vi "Gyro Signal 3-Axis Display from other MCU.vi"() -> ()   [LabVIEW 2015]
uses:
  <vilib>/Utility/error.llb/DialogType.ctl
  <vilib>/Instr/_visa.llb/VISA Configure Serial Port (Instr).vi
panel:
  out "System Time":dbl
  in  "Stop Button":bool
  out "Z-Array":dbl[](array[numeric])
  out "Y-Array":dbl[](array[numeric])
  out "X-Array":dbl[](array[numeric])
  out "Gyro Reading Z":dbl(knob) scale=-250.0..250.0
  out "Gyro Reading Y":dbl(knob) scale=-250.0..250.0
  out "Data Buffer":u8[](array[numeric])
  in  "parity (0:none)":enum16{"None", "Odd", "Even", "Mark", "Space"}(ring)
  out "Gyro Reading X":dbl(knob) scale=-250.0..250.0
  in  "VISA resource name":refnum<visa-resource-name>="COM5"
  in  "Stop bits (1 bit)":u16(ring)=10 items=["1.0"=10, "1.5"=15, "2.0"=20]
  in  "Baud rate":u32=115200
  # "Setup of Basic Serial Coms"
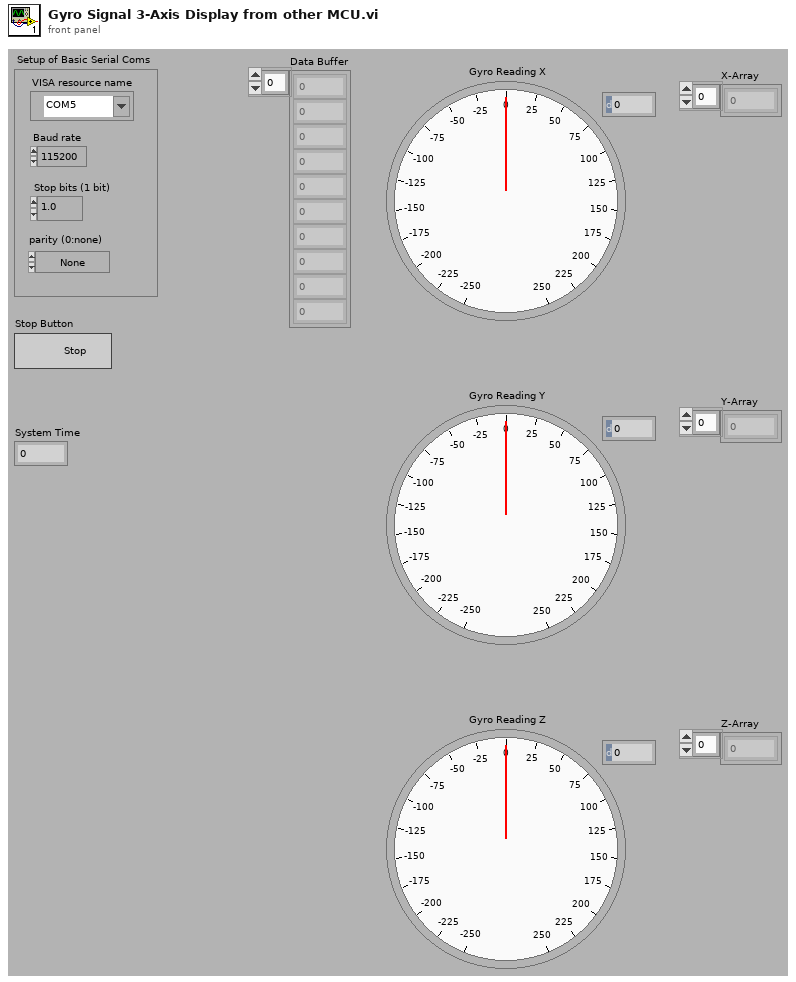
[diagram p1: front panel]
types:
  T1 = typedef "DialogType.ctl" = u16
  T2 = cluster{"Data Buffer[0]":u8, "Data Buffer[1]":u8, "Data Buffer[2]":u8, "Data Buffer[3]":u8, "Data Buffer[4]":u8, "Data Buffer[5]":u8, "Data Buffer[6]":u8, "Data Buffer[7]":u8, "Data Buffer[8]":u8, "Data Buffer[9]":u8}
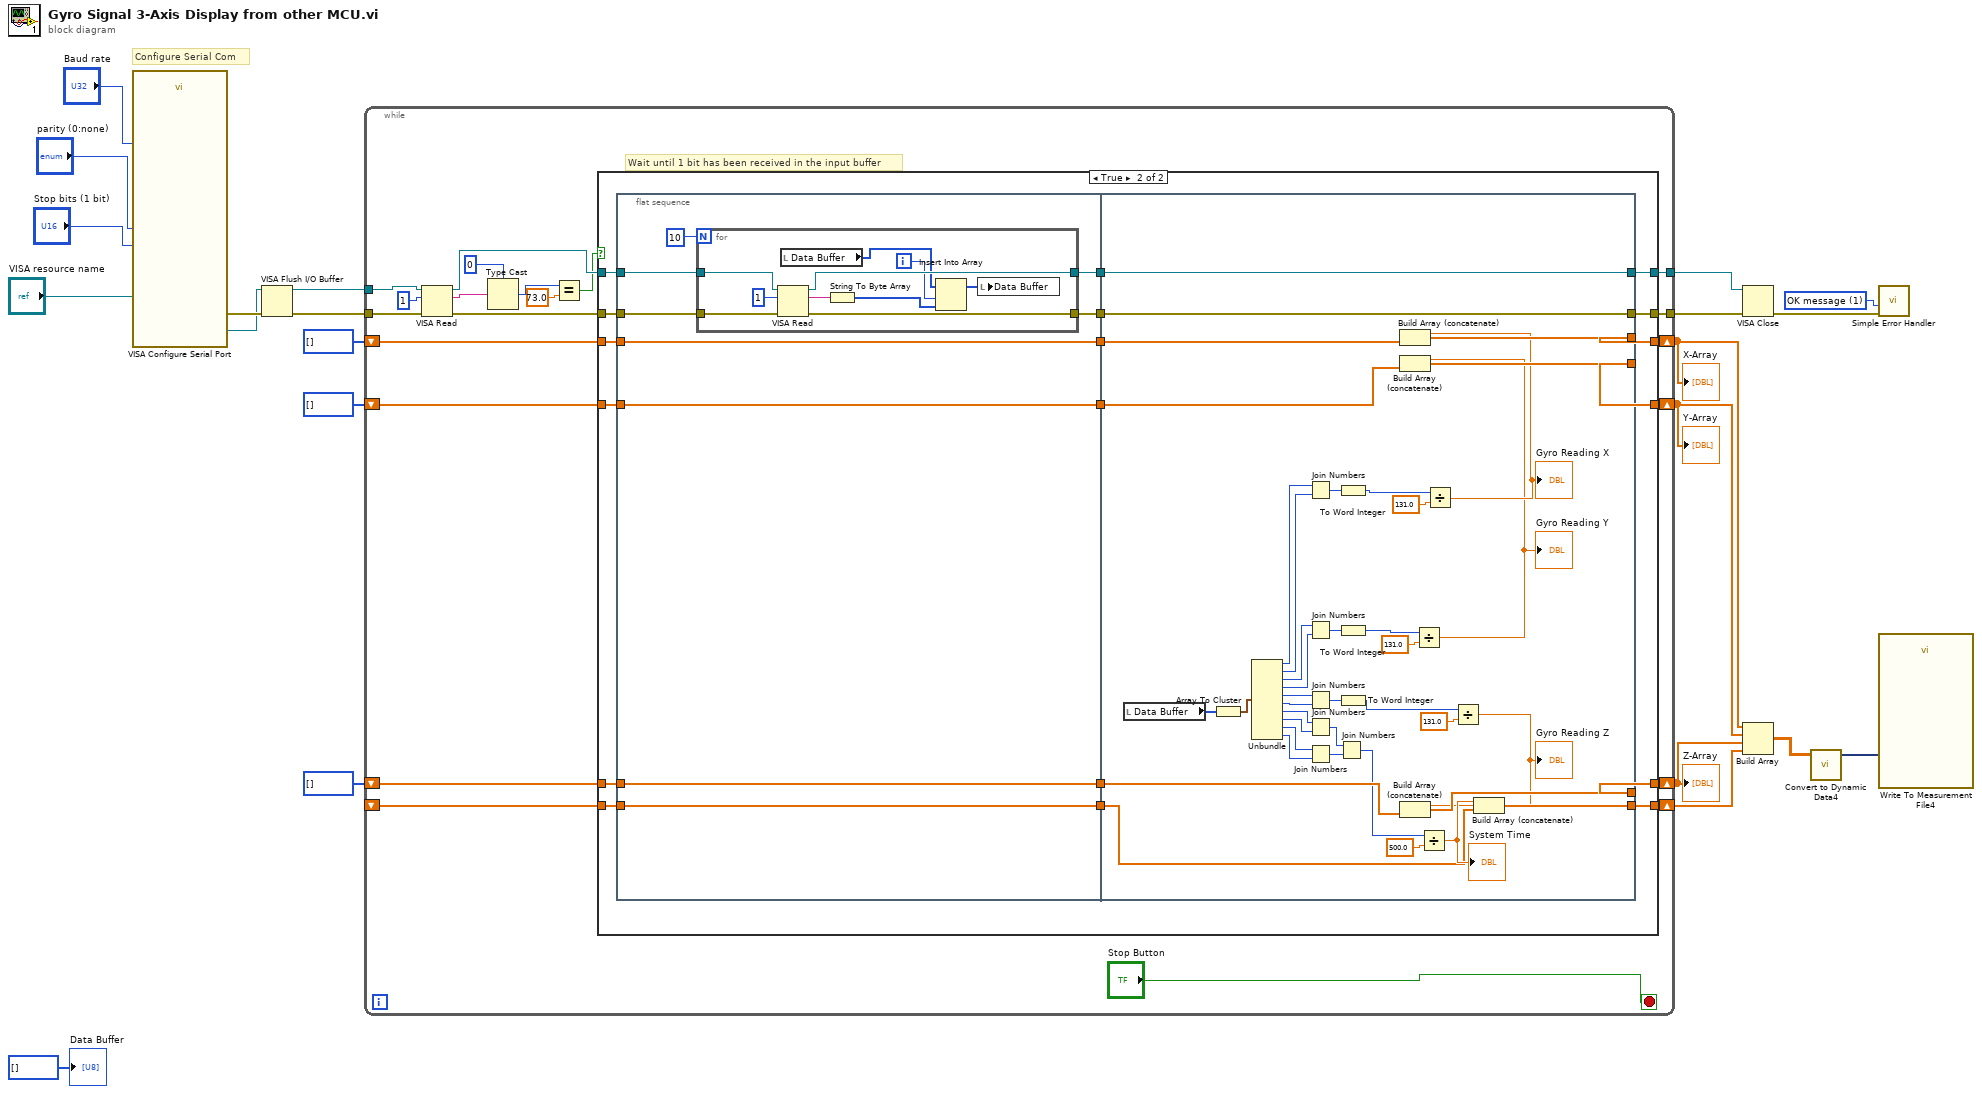
[diagram p0: block diagram]
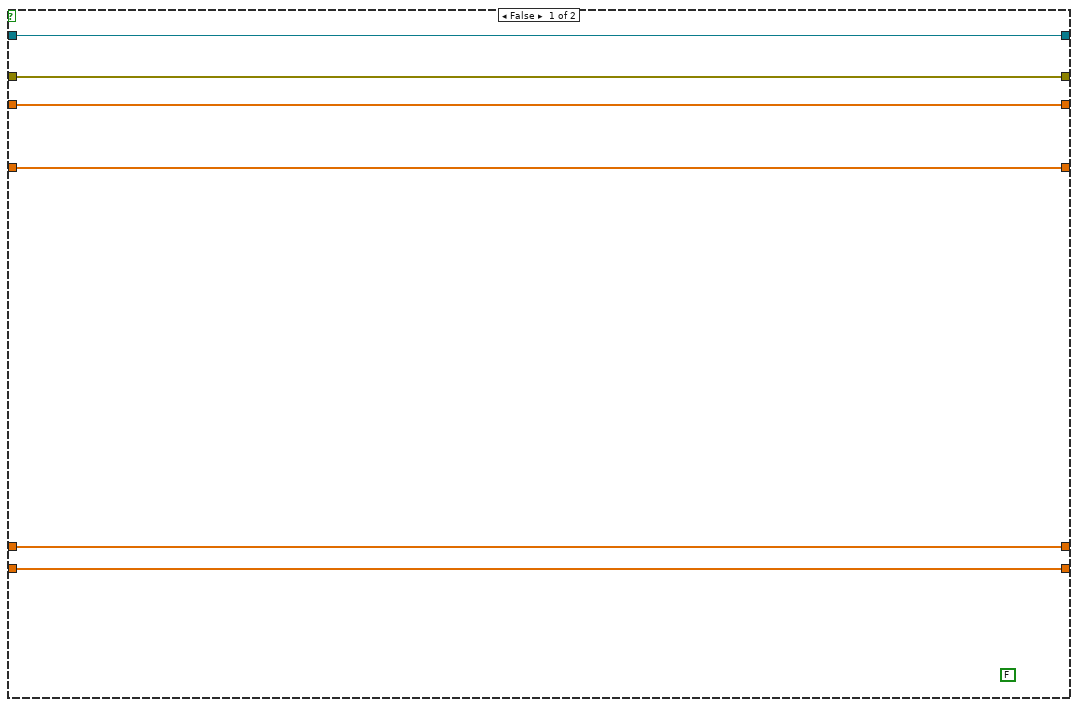
[diagram p2: hidden frame]
diagram:
  w18 = T1 1 items=["no dialog", "OK message", "continue or stop message", "OK message + warnings", "continue/stop + warnings"] ("type of dialog (OK msg:1)")
  # "Configure Serial Com"
  n1 = call-poly "VISA Configure Serial Port"("VISA resource name"="VISA resource name", "baud rate (9600)"="Baud rate", "parity (0:none)"="parity (0:none)", "stop bits (10: 1 bit)"="Stop bits (1 bit)") -> ("VISA resource name out"=w16:refnum<visa-resource-name>, "error out"=w17:errorcluster)  [unwired: 10 in]
  n2 = VISA Flush I/O Buffer(VISA resource name=w16, error in (no error)=w17) -> (VISA resource name out=w15:refnum<visa-resource-name>, error out=w14:errorcluster)  [unwired: 1 in]
  n3 = while {
    tunnel: w15 -> [w35]
    tunnel: w14 -> [w34]
    tunnel: [w43] -> w12
    tunnel: [w42] -> w11
    shift-right: [w41] -> w4
    shift-left: i16[] [] -> [w40]
    shift-right: [w36] -> w3
    shift-left: i16[] [] -> [w37]
    shift-right: [w39] -> w2
    shift-left: i16[] [] -> [w38]
    shift-right: [w25] -> w1
    shift-left: _ -> [w24]
    stop <- "Stop Button" stop-if-true
    # "Wait until 1 bit has been received in the input buffer"
    n4 = VISA Read(VISA resource name=w35, byte count=u32 1, error in (no error)=w34) -> (VISA resource name out=w32:refnum<visa-resource-name>, read buffer=w26:string, error out=w31:errorcluster)  [unwired: 1 out]
    n5 = Type Cast(type=u8 0, x=w26) -> (*(type *) &x=w29:u8)
    n6 = Equal?(x=w29, y=73.0) -> (x = y?=w27:bool)
    n7 = case shown="True" w27 {
      tunnel: [w46 w65] -> w43
      tunnel: [w45 w64] -> w42
      tunnel: [w49 w63] -> w41
      tunnel: w40 -> [w49 w62]
      tunnel: [w48 w60] -> w39
      tunnel: w38 -> [w48 w59]
      tunnel: w37 -> [w47 w57]
      tunnel: [w47 w55] -> w36
      tunnel: w32 -> [w46 w54]
      tunnel: w31 -> [w45 w53]
      tunnel: [w44 w52] -> w25
      tunnel: w24 -> [w44 w51]
      frame False {
        (unwired) FALSE ("LIMIT ERROR")
      }
      frame True {
        n8 = flat-sequence {
          tunnel: [w75] -> w67
          tunnel: [w74] -> w66
          tunnel: w62 -> [w73]
          tunnel: [w73] -> w61
          tunnel: w59 -> [w72]
          tunnel: [w72] -> w58
          tunnel: w57 -> [w71]
          tunnel: [w71] -> w56
          tunnel: w54 -> [w70]
          tunnel: w53 -> [w69]
          tunnel: w51 -> [w68]
          tunnel: [w68] -> w50
          tunnel: w67 -> [w117]
          tunnel: w66 -> [w116]
          tunnel: [w117] -> w65
          tunnel: [w116] -> w64
          tunnel: [w112] -> w63
          tunnel: w61 -> [w111]
          tunnel: [w110] -> w60
          tunnel: w58 -> [w109]
          tunnel: w56 -> [w108]
          tunnel: [w107] -> w55
          tunnel: [w98] -> w52
          tunnel: w50 -> [w97]
          frame #0 {
            n9 = for {
              N: 10 -> [_]
              tunnel: [w85] -> w75
              tunnel: [w84] -> w74
              tunnel: w70 -> [w78]
              tunnel: w69 -> [w77]
              i -> [w79]
              n10 = VISA Read(VISA resource name=w78, byte count=u32 1, error in (no error)=w77) -> (VISA resource name out=w85:refnum<visa-resource-name>, read buffer=w83:string, error out=w84:errorcluster)  [unwired: 1 out]
              n11 = local read "Data Buffer"() -> (w81:u8[])
              n12 = String To Byte Array(string=w83) -> (unsigned byte array=w82:u8[])
              n13 = Insert Into Array(array=w81, index=w79, new element=w82) -> (w80:u8[])
              n14 = local write "Data Buffer"(w80) -> ()
            }
          }
          frame #1 {
            n15 = local read "Data Buffer"() -> (w125:u8[])
            n16 = Array To Cluster(array=w125) -> (cluster=w123:T2)
            n17 = Unbundle(w123) -> ("Data Buffer[0]"=w121:u8, "Data Buffer[1]"=w120:u8, "Data Buffer[2]"=w119:u8, "Data Buffer[3]"=w118:u8, "Data Buffer[4]"=w114:u8, "Data Buffer[5]"=w113:u8, "Data Buffer[6]"=w104:u8, "Data Buffer[7]"=w103:u8, "Data Buffer[8]"=w102:u8, "Data Buffer[9]"=w101:u8)
            n18 = Join Numbers(hi=w121, lo=w120) -> ((hi.lo)=w124:u16)
            n19 = Join Numbers(hi=w119, lo=w118) -> ((hi.lo)=w122:u16)
            n20 = Join Numbers(hi=w114, lo=w113) -> ((hi.lo)=w115:u16)
            n21 = Join Numbers(hi=w104, lo=w103) -> ((hi.lo)=w106:u16)
            n22 = Join Numbers(hi=w102, lo=w101) -> ((hi.lo)=w105:u16)
            n23 = Join Numbers(hi=w106, lo=w105) -> ((hi.lo)=w96:u32)
            n24 = To Word Integer(number=w124) -> (16bit integer=w92:i16)
            n25 = To Word Integer(number=w122) -> (16bit integer=w91:i16)
            n26 = To Word Integer(number=w115) -> (16bit integer=w88:i16)
            n27 = Divide(x=w91, y=131.0) -> (x/y=w90:dbl)
            "Gyro Reading Y" <- w90
            n28 = Build Array (concatenate)(w90, w108) -> (w107:dbl[])
            n29 = Divide(x=w96, y=500.0) -> (x/y=w99:dbl)
            "System Time" <- w99
            n30 = Divide(x=w92, y=131.0) -> (x/y=w93:dbl)
            "Gyro Reading X" <- w93
            n31 = Build Array (concatenate)(w93, w111) -> (w112:dbl[])
            n32 = Divide(x=w88, y=131.0) -> (x/y=w89:dbl)
            "Gyro Reading Z" <- w89
            n33 = Build Array (concatenate)(w89, w109) -> (w110:dbl[])
            n34 = Build Array (concatenate)(w99, w97) -> (w98:dbl[])
          }
        }
      }
    }
  }
  "X-Array" <- w4
  "Y-Array" <- w3
  "Z-Array" <- w2
  n35 = VISA Close(VISA resource name=w12, error in (no error)=w11) -> (error out=w19:errorcluster)
  n36 = Build Array(w4, w3, w2, w1) -> (w6:dbl[][])
  n37 = call "Convert to Dynamic Data4"("2D Array"=w6) -> ("Dynamic Data Type"=w5:dynamicdata)  [unwired: 3 in]
  n38 = call <vilib>:"Simple Error Handler.vi"("type of dialog (OK msg:1)"=w18, "error in (no error)"=w19) -> ()  [unwired: 3 in, 5 out]
  n39 = call "Write To Measurement File4"("Signals"=w5) -> ()  [unwired: 16 in, 3 out]
  "Data Buffer" <- u8[] [] ("Data Buffer")
